vi "SetDataEventStreamBlock.vi"(8 "error in (no error)":errorcluster, 10 "block":i32, 11 "data event reference":T1) -> (0 "error out":errorcluster)   [LabVIEW 2017, in "DataEvent.lvlib"]
uses:
  <vilib>/addons/InsightCM/Devices/Shared/Common/DataEvent/DataEvent.lvlib
  <vilib>/addons/InsightCM/Devices/Shared/Common/DataEvent/controls/EventReference.ctl
  <vilib>/addons/InsightCM/Devices/Shared/Common/DataEvent/controls/Event.ctl
  <vilib>/addons/InsightCM/MessageBus/Base/controls/DataEvent.ctl
  <vilib>/addons/InsightCM/MessageBus/Base/controls/KeyValuePair.ctl
  <vilib>/addons/InsightCM/Devices/Shared/Common/DataEvent/controls/DataSet.ctl
  <vilib>/addons/InsightCM/MessageBus/Base/controls/DataSetMetadata.ctl
  <vilib>/addons/InsightCM/MessageBus/Base/controls/TrendPoint.ctl
  <vilib>/addons/InsightCM/MessageBus/Base/controls/TrendAlarmUpdate.ctl
  <vilib>/addons/InsightCM/MessageBus/Base/controls/TrendAlarmTransition.ctl
  <vilib>/addons/InsightCM/Utilities/PropertyHelpers/PropertyHelpers.lvlib
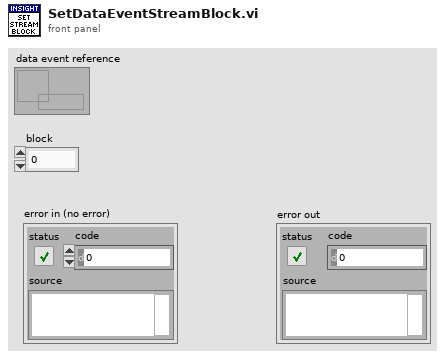
[diagram p1: front panel]
types:
  T1 = typedef "DataEvent.lvlib/EventReference.ctl" = refnum<data-value>
  T2 = typedef "DataEvent.lvlib/Event.ctl" = cluster{"DataEvent":T3, "DataSets":T5[], "TrendPoints":T7[], "Alarms":T8[]}
  T3 = typedef "DataEvent.ctl" = cluster{"Id":string, "AssetNodeId":string, "Timestamp":i64, "Props":T4[]}
  T4 = typedef "KeyValuePair.ctl" = cluster{"Key":string, "Value":string}
  T5 = typedef "DataEvent.lvlib/DataSet.ctl" = cluster{"DataSetMetadata":T6, "Values":sgl[], "Values DVR":refnum<data-value>}
  T6 = typedef "DataSetMetadata.ctl" = cluster{"Id":string, "DataEventId":string, "AssetNodeId":string, "Type":string, "T0":i64, "Props":T4[]}
  T7 = typedef "TrendPoint.ctl" = cluster{"TrendPointId":string, "DataEventId":string, "Timestamp":i64, "Value":dbl, "Props":T4[]}
  T8 = typedef "TrendAlarmUpdate.ctl" = cluster{"RuleId":string, "Transition":T9}
  T9 = typedef "TrendAlarmTransition.ctl" = cluster{"At":i64, "Severity":i32, "Value":dbl}
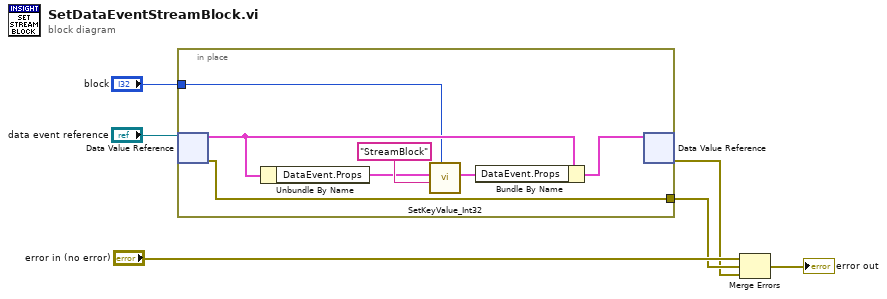
[diagram p0: block diagram]
diagram:
  n1 = in-place {
    in-place-border: "block" -> [w10]
    in-place-border: [w7] -> w3
    n2 = in-place-dvr #1("data event reference") -> (w12:T2, w7:errorcluster)
    n3 = Unbundle By Name(w12) -> ("DataEvent.Props"=w9:T4[])
    n4 = call <vilib>:"SetKeyValue_Int32.vi"("value"=w10, "key"="StreamBlock", "key value pairs"=w9) -> ("key value pairs out"=w8:T4[])  [unwired: 8 in]
    n5 = Bundle By Name(cluster=w12, "DataEvent.Props"=w8) -> (w11:T2)
    n6 = in-place-dvr #1(w11) -> (w2:errorcluster)  [unwired: 1 out]
  }
  n7 = Merge Errors("error in (no error)", w3, w2) -> (→"error out":errorcluster)
